vi "Table, Get Data Dimensions.vi"(8 "error in":errorcluster, 11 "Tbl Refnum":refnum<vi>) -> (0 "error out":errorcluster, 1 "col_n":i32=-1, 2 "row_n":i32=-1, 3 "Tbl Refnum out":refnum<vi>)   [LabVIEW 2010]
doc: "Gets table data array number of row and column elements."
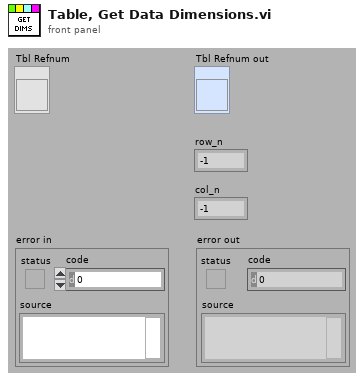
[diagram p1: front panel]
types:
  T1 = cluster{"[0]":i32, "[1]":i32, "[2]":i32, "[3]":i32, "[4]":i32, "[5]":i32, "[6]":i32, "[7]":i32, "[8]":i32}
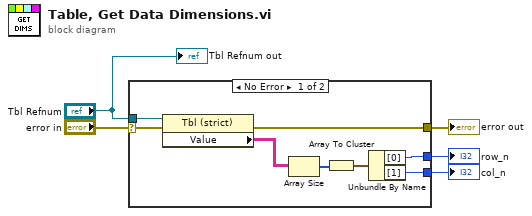
[diagram p0: block diagram]
diagram:
  n1 = case shown="No Error" "error in" {
    selector: "error in" -> [w6 w14]
    tunnel: "Tbl Refnum" -> [w13 _]
    tunnel: [w9 _] -> w4
    tunnel: [w8 _] -> w3
    tunnel: [w7 w14] -> w2
    frame No Error {
      n2 = property class="Tbl (strict)"(reference=w13, error in=w6) -> (error out=w7:errorcluster, "Value"=w12:string[][])  [unwired: 1 out]
      n3 = Array Size(array=w12) -> (size(s)=w11:i32[])
      n4 = Array To Cluster(array=w11) -> (cluster=w10:T1)
      n5 = Unbundle By Name(w10) -> ("[0]"=w9:i32, "[1]"=w8:i32)
    }
    frame Error {
    }
  }
  "col_n" <- w3
  "row_n" <- w4
  "error out" <- w2
  "Tbl Refnum out" <- "Tbl Refnum"
